vi "LED分析仪全部数据.vi"(8 "error in (no error)":errorcluster caption="错误输入（无错误）", 10 "地址":string="02", 11 "MyIndex":u8) -> (0 "error out":errorcluster caption="错误输出", 3 "亮度":u32[](array[numeric]))   [LabVIEW 2015]
uses:
  <vilib>/Instr/_visa.llb/VISA Configure Serial Port (Instr).vi
panel:
  out "长度":i32
  out "所有数据":u16[][](array[numeric])
  out "Read":string
  out "Send":string
  # "R"
  # "G"
  # "B"
  # "i"
  # "H"
  # "S"
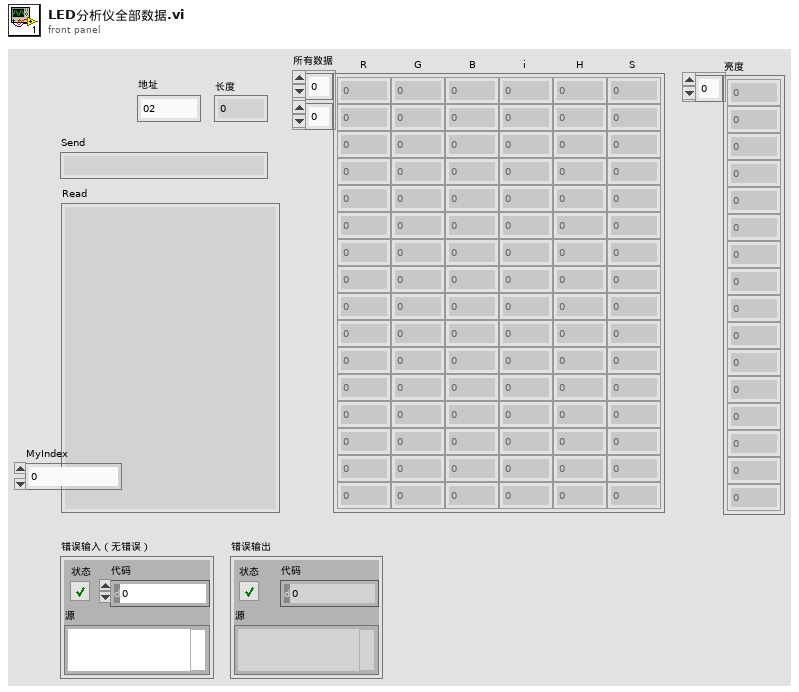
[diagram p1: front panel]
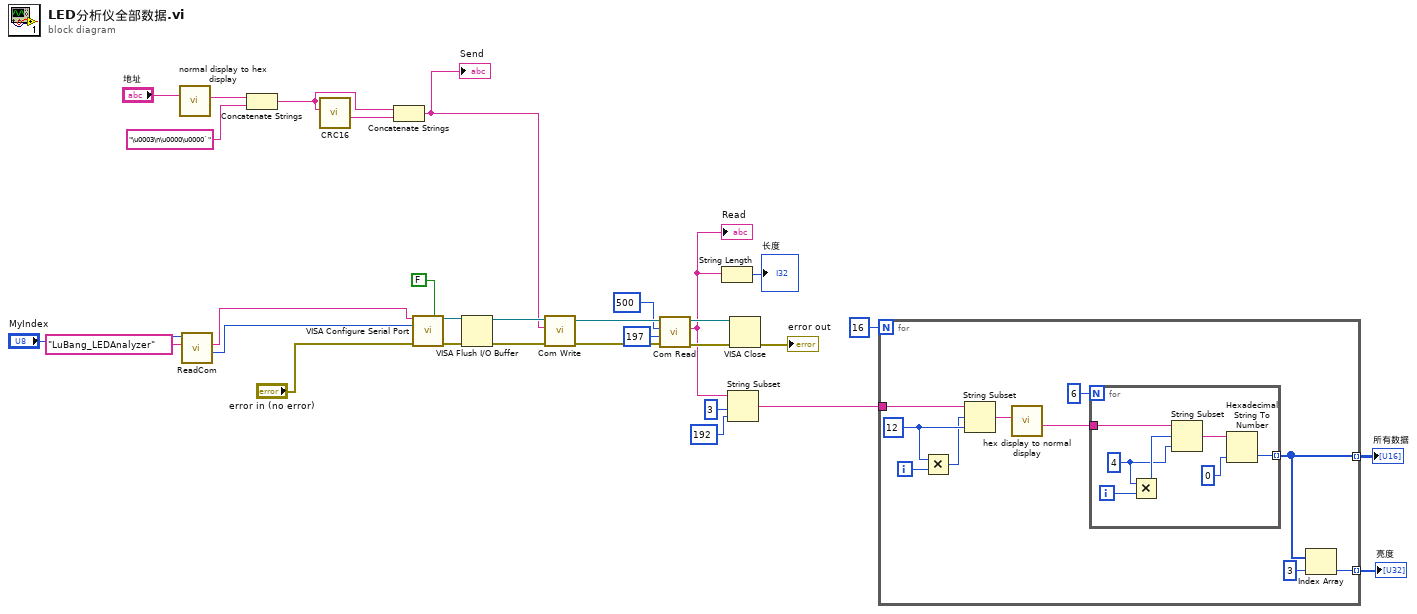
[diagram p0: block diagram]
diagram:
  n1 = call "normal display to hex display.vi"("Normal display"="地址") -> ("Hex display"=w23:string)  [unwired: 6 in]
  n2 = call "ReadCom.vi"("仪器名称"="LuBang_LEDAnalyzer", "MyIndex"="MyIndex") -> ("Baudrate"=w1:i32, "COM"=w2:string)  [unwired: 7 in, 1 out]
  n3 = Concatenate Strings(w23, "\u0003\n\u0000\u0000`") -> (w27:string)
  n4 = call "CRC16.vi"("输入字符串"=w27) -> ("CRC16(String)"=w26:string)  [unwired: 9 in, 1 out]
  n5 = Concatenate Strings(w27, w26) -> (w20:string)
  "Send" <- w20
  n6 = call-poly "VISA Configure Serial Port"("VISA resource name"=w2, "Enable Termination\nChar (T)"=FALSE ("Enable Termination\nChar (T)"), "baud rate (9600)"=w1, "error in (no error)"="error in (no error)") -> ("VISA resource name out"=w28:refnum<visa-resource-name>, "error out"=w29:errorcluster)  [unwired: 10 in]
  n7 = VISA Flush I/O Buffer(VISA resource name=w28, error in (no error)=w29) -> (VISA resource name out=w22:refnum<visa-resource-name>, error out=w21:errorcluster)  [unwired: 1 in]
  n8 = call "Com Write.vi"("错误输入（无错误）"=w21, "Wbuff"=w20, "VISA In"=w22) -> ("错误输出"=w19:errorcluster, "VISA Out"=w18:refnum<visa-resource-name>)  [unwired: 7 in]
  n9 = call "Com Read.vi"("错误输入（无错误）"=w19, "num"=u32 197, "超时"=u32 500, "VISA In"=w18) -> ("错误输出"=w14:errorcluster, "buff"=w6:string, "VISA Out"=w15:refnum<visa-resource-name>)  [unwired: 5 in]
  "Read" <- w6
  n10 = String Length(string=w6) -> (length=→"长度":i32)
  n11 = String Subset(string=w6, offset (0)=3 ("长度（剩余）"), length (rest)=192 ("长度（剩余）")) -> (substring=w10:string)
  n12 = VISA Close(VISA resource name=w15, error in (no error)=w14) -> (error out=→"error out":errorcluster)
  n13 = for {
    N: 16 -> [_]
    tunnel: w10 -> [w40]
    tunnel: [w34] -> w8 mode=indexing
    tunnel: [w32] -> w7 mode=indexing
    i -> [w39]
    w38 = 12 ("长度（剩余）")
    n14 = Multiply(x=w38, y=w39) -> (x*y=w37:i32)
    n15 = String Subset(string=w40, offset (0)=w37, length (rest)=w38) -> (substring=w36:string)
    n16 = call "hex display to normal display.vi"("Hex display"=w36) -> ("Normal display"=w35:string)  [unwired: 10 in]
    n17 = for {
      N: 6 -> [_]
      tunnel: w35 -> [w48]
      tunnel: [w43] -> w34 mode=indexing
      i -> [w47]
      w45 = 4
      n18 = Multiply(x=w45, y=w47) -> (x*y=w46:i32)
      n19 = String Subset(string=w48, offset (0)=w46, length (rest)=w45) -> (substring=w44:string)
      n20 = Hexadecimal String To Number(string=w44, default (0uL)=u32 0) -> (number=w43:u32)  [unwired: 1 in, 1 out]
    }
    n21 = Index Array(array=w34, index=3 ("索引")) -> (element=w32:u32)
  }
  "所有数据" <- w8
  "亮度" <- w7
